vi "Serialize Object (XML).vi"(8 "error in":errorcluster, 11 "object in":refnum<class "_ISerializable.lvclass">) -> (0 "error out":errorcluster, 1 "key-value-type":T1[](array[typedef]), 3 "dup object":refnum<class "_ISerializable.lvclass">, 4 "values":string[](array[string]), 6 "names":string[](array[string]))   [LabVIEW 2018, in "Serializer.lvclass"]
uses:
  Serializer.lvclass
  _Serializable Base Object/_ISerializable.lvclass
  Typedefs/key-value-type cluster.ctl
  <vilib>/xml/Close Reference(Node).vi
  <vilib>/xml/NI_XML.lvlib
  <resource>/objmgr/DOMUserDefRef.rc
panel:
  out "type":string[](array[string])
  out "object xml string":string
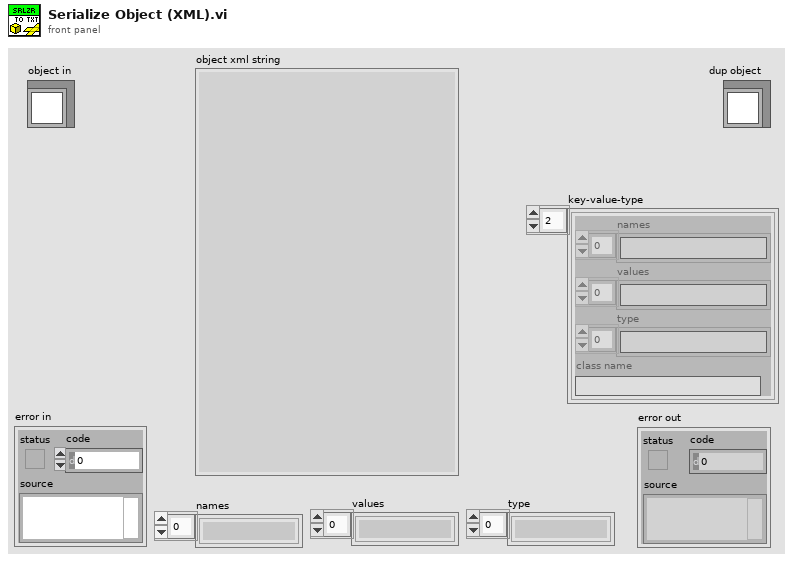
[diagram p1: front panel]
types:
  T1 = typedef "key-value-type cluster.ctl" = cluster{"names":string[], "values":string[], "type":string[], "class name":string}
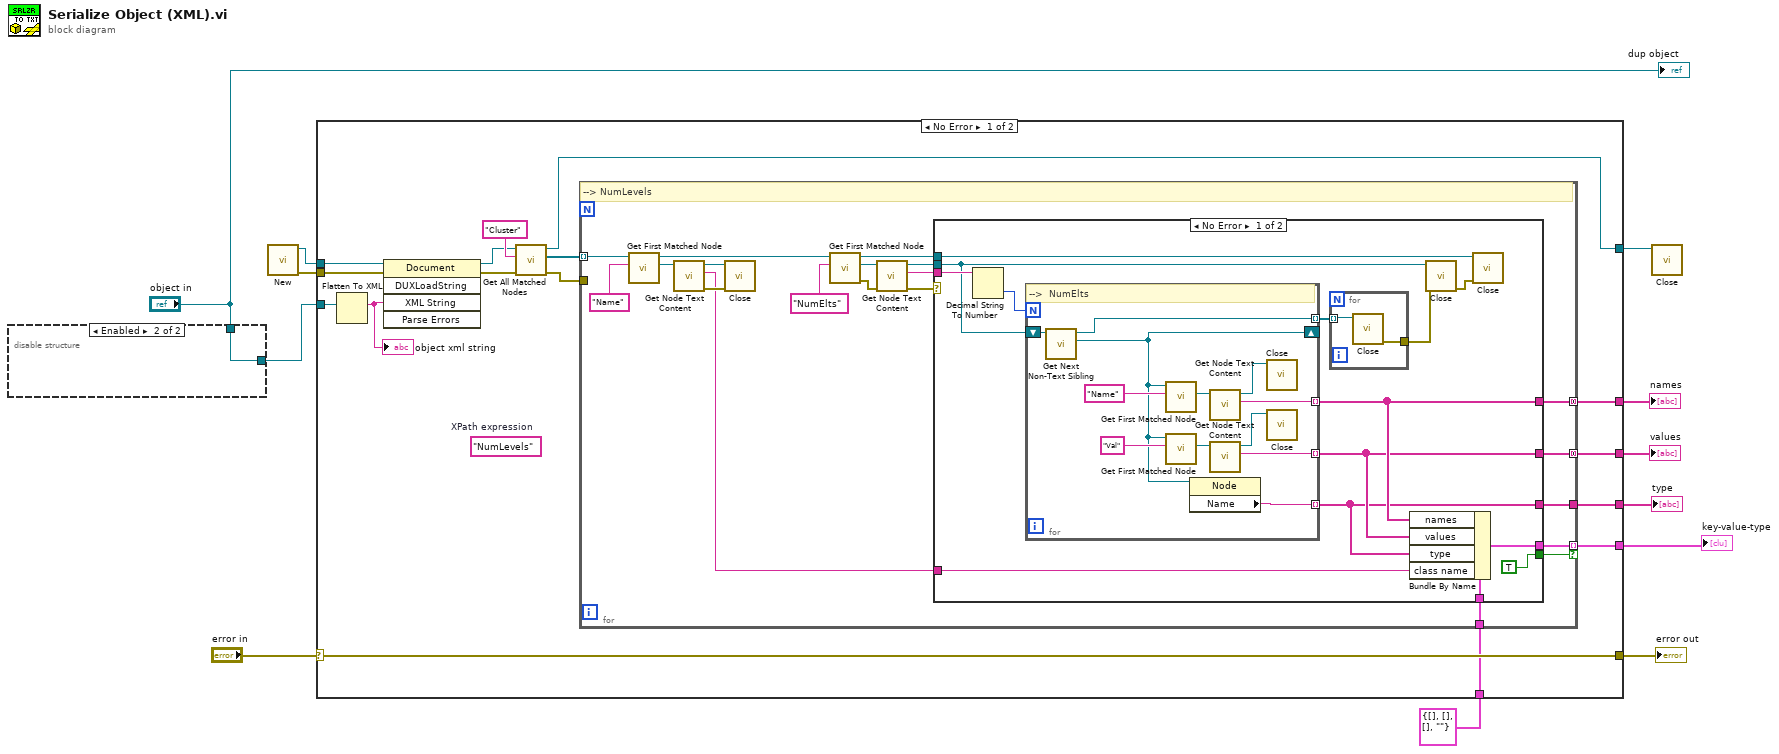
[diagram p0: block diagram]
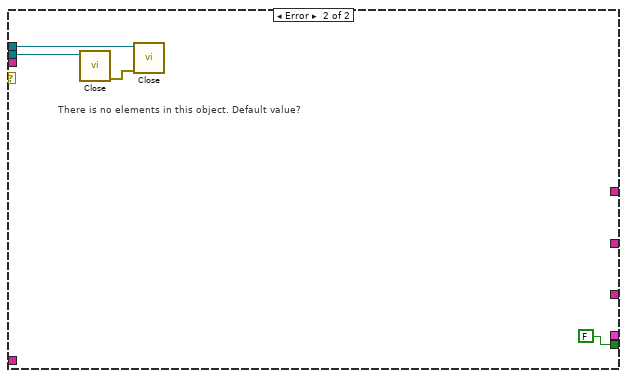
[diagram p2: hidden frame]
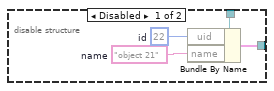
[diagram p4: hidden frame]
diagram:
  n1 = disable-structure shown="Enabled" {
    disable-tunnel: "object in" -> [w14 w17]
    disable-tunnel: [w13 w17] -> w10
    frame Disabled {
      w15 = "object 21"  # name
      w16 = 22  # id
      n2 = Bundle By Name(cluster=w14, "uid"=w16, "name"=w15) -> (w13:cluster{})
    }
    frame Enabled {
    }
  }
  n3 = call <vilib>:"New.vi"() -> ("error out"=w9:errorcluster, "DOM document out"=w8:refnum<k20>)  [unwired: 8 in]
  n4 = case shown="No Error" "error in" {
    selector: "error in" -> [w33 w87]
    tunnel: [w33 w87] -> w11
    tunnel: w10 -> [w32 _]
    tunnel: w9 -> [w30 _]
    tunnel: w8 -> [w29 w86]
    tunnel: [w25 w86] -> w7
    tunnel: [w24 _] -> w6
    tunnel: [w23 _] -> w5
    tunnel: [w20 _] -> w3
    tunnel: T1 {"names"=[], "values"=[], "type"=[], "class name"=""} -> [w19 _]
    tunnel: [w18 _] -> w1
    frame No Error {
      (unwired) "NumLevels"  # XPath expression
      n5 = Flatten To XML(anything=w32) -> (xml string=w28:string)
      "object xml string" <- w28
      n6 = invoke class="Document" method="DUXLoadString"(reference=w29, error in=w30, "XML String"=w28) -> (reference out=w22:refnum<k20>, error out=w27:errorcluster)  [unwired: 2 in, 3 out]
      n7 = call <vilib>:"Get All Matched Nodes.vi"("error in (no error)"=w27, "XPath expression"="Cluster", "node in"=w22) -> ("error out"=w26:errorcluster, "node result array"=w21:refnum<k20>[], "node out"=w25:refnum<k20>)  [unwired: 6 in]
      n8 = for {
        tunnel: w26 -> [_]
        tunnel: [w46] -> w24 mode=concatenating
        tunnel: [w45] -> w23 mode=concatenating
        tunnel: w21 -> [w39] mode=indexing
        tunnel: [w44] -> w20
        tunnel: w19 -> [w43]
        tunnel: [w42] -> w18 mode=indexing if=w41
        # "--> NumLevels"
        n9 = call <vilib>:"Get First Matched Node.vi"("XPath expression"="Name", "node in"=w39) -> ("node result"=w37:refnum<k20>, "node out"=w38:refnum<k20>)  [unwired: 7 in, 1 out]
        n10 = call <vilib>:"Get Node Text Content.vi"("node in"=w37) -> ("error out"=w35:errorcluster, "node text"=w34:string, "node out"=w36:refnum<k20>)  [unwired: 8 in]
        n11 = call-poly <vilib>:"Close.vi"("error in (no error)"=w35, "node"=w36) -> ()  [unwired: 7 in, 1 out]
        n12 = call <vilib>:"Get First Matched Node.vi"("XPath expression"="NumElts", "node in"=w38) -> ("error out"=w48:errorcluster, "node result"=w52:refnum<k20>, "node out"=w49:refnum<k20>)  [unwired: 7 in]
        n13 = call <vilib>:"Get Node Text Content.vi"("error in (no error)"=w48, "node in"=w52) -> ("error out"=w47:errorcluster, "node text"=w51:string, "node out"=w50:refnum<k20>)  [unwired: 7 in]
        n14 = case shown="No Error" w47 {
          tunnel: w51 -> [w67 _]
          tunnel: w50 -> [w61 w85]
          tunnel: w49 -> [w66 w84]
          tunnel: [w58 _] -> w46
          tunnel: [w57 _] -> w45
          tunnel: [w56 _] -> w44
          tunnel: w43 -> [w60 _]
          tunnel: [w59 _] -> w42
          tunnel: [TRUE FALSE] -> w41
          tunnel: w34 -> [w54 _]
          frame No Error {
            n15 = Decimal String To Number(string=w67) -> (number=w65:i32)  [unwired: 2 in, 1 out]
            n16 = for {
              N: w65 -> [_]
              shift-right: [w71] -> _
              shift-left: w61 -> [w81]
              tunnel: [w78] -> w58 mode=indexing
              tunnel: [w77] -> w57 mode=indexing
              tunnel: [w72] -> w63 mode=indexing
              tunnel: [w70] -> w56 mode=indexing
              # "-->  NumElts"
              n17 = call <vilib>:"Get Next Non-Text Sibling.vi"("node in"=w81) -> ("sibling node"=w71:refnum<k20>, "node out"=w72:refnum<k20>)  [unwired: 7 in, 2 out]
              n18 = call <vilib>:"Get First Matched Node.vi"("XPath expression"="Name", "node in"=w71) -> ("node result"=w76:refnum<k20>)  [unwired: 7 in, 2 out]
              n19 = call <vilib>:"Get First Matched Node.vi"("XPath expression"="Val", "node in"=w71) -> ("node result"=w75:refnum<k20>)  [unwired: 7 in, 2 out]
              n20 = property class="Node"(reference=w71) -> ("Name"=w70:string)  [unwired: 1 in, 2 out]
              n21 = call <vilib>:"Get Node Text Content.vi"("node in"=w76) -> ("node text"=w78:string, "node out"=w74:refnum<k20>)  [unwired: 8 in, 1 out]
              n22 = call <vilib>:"Get Node Text Content.vi"("node in"=w75) -> ("node text"=w77:string, "node out"=w73:refnum<k20>)  [unwired: 8 in, 1 out]
              n23 = call-poly <vilib>:"Close.vi"("node"=w74) -> ()  [unwired: 8 in, 1 out]
              n24 = call-poly <vilib>:"Close.vi"("node"=w73) -> ()  [unwired: 8 in, 1 out]
            }
            n25 = for {
              tunnel: w63 -> [w69] mode=indexing
              tunnel: [w68] -> w62
              n26 = call-poly <vilib>:"Close.vi"("node"=w69) -> ("error out"=w68:errorcluster)  [unwired: 8 in]
            }
            n27 = Bundle By Name(cluster=w60, "names"=w58, "values"=w57, "type"=w56, "class name"=w54) -> (w59:T1)
            n28 = call-poly <vilib>:"Close.vi"("error in (no error)"=w62, "node"=w61) -> ("error out"=w64:errorcluster)  [unwired: 7 in]
            n29 = call-poly <vilib>:"Close.vi"("error in (no error)"=w64, "node"=w66) -> ()  [unwired: 7 in, 1 out]
          }
          frame Error {
            # "There is no elements in this object. Default value?"
            n30 = call-poly <vilib>:"Close.vi"("node"=w85) -> ("error out"=w83:errorcluster)  [unwired: 8 in]
            n31 = call-poly <vilib>:"Close.vi"("error in (no error)"=w83, "node"=w84) -> ()  [unwired: 7 in, 1 out]
          }
        }
      }
    }
    frame Error {
    }
  }
  "error out" <- w11
  "values" <- w5
  "names" <- w6
  "type" <- w3
  "key-value-type" <- w1
  n32 = call-poly <vilib>:"Close.vi"("node"=w7) -> ()  [unwired: 8 in, 1 out]
  "dup object" <- "object in"
